vi "GetFileVersionProperties.vi"() -> (3 "properties":T1[](array[typedef]))   [LabVIEW 2017, in "Tdms.lvlib"]
uses:
  <vilib>/addons/InsightCM/Utilities/Tdms/Tdms.lvlib
  <vilib>/addons/InsightCM/Utilities/Tdms/controls/Property.ctl
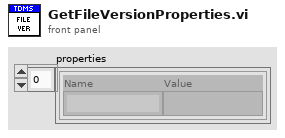
[diagram p1: front panel]
types:
  T1 = typedef "Tdms.lvlib/Property.ctl" = cluster{"Name":string, "Value":variant}
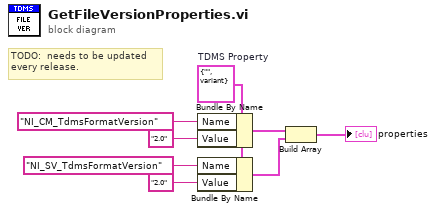
[diagram p0: block diagram]
diagram:
  w3 = T1 {"Name"="", "Value"=variant}  # TDMS Property
  # "TODO:  needs to be updated\nevery release."
  n1 = Bundle By Name(cluster=w3, "Name"="NI_CM_TdmsFormatVersion", "Value"="2.0" ("Name")) -> (w6:T1)
  n2 = Bundle By Name(cluster=w3, "Name"="NI_SV_TdmsFormatVersion", "Value"="2.0" ("Name")) -> (w7:T1)
  n3 = Build Array(w6, w7) -> (→"properties":T1[])
